vi "customise_left_slider.vi"(8 "error in":errorcluster, 11 "slide_left_ref":refnum<vi>) -> (0 "error out":errorcluster)   [LabVIEW 2020]
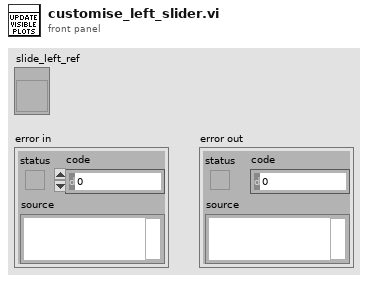
[diagram p1: front panel]
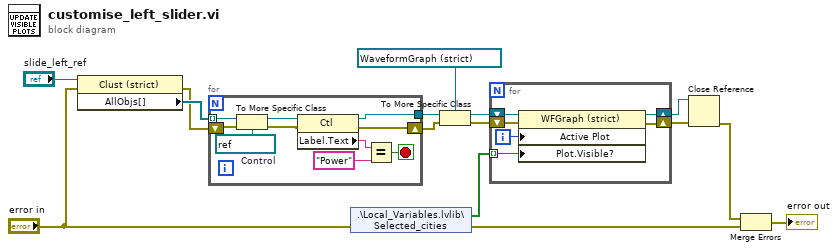
[diagram p0: block diagram]
diagram:
  n1 = property class="Clust (strict)"(reference="slide_left_ref", error in="error in") -> (error out=w2:errorcluster, "AllObjs[]"=w4:refnum<vi>[])  [unwired: 1 out]
  n2 = for {
    tunnel: w4 -> [w25] mode=indexing
    tunnel: [w19] -> w3
    shift-right: [w16] -> w1
    shift-left: w2 -> [w18]
    stop <- w20 stop-if-true
    w23 = refnum<vi> refnum  # Control
    n3 = To More Specific Class(target class=w23, reference=w25, error in=w18) -> (specific class reference=w24:refnum<vi>, error out=w17:errorcluster)
    n4 = property class="Ctl"(reference=w24, error in=w17) -> (reference out=w19:refnum<vi>, error out=w16:errorcluster, "Label.Text"=w22:string)
    n5 = Equal?(x=w22, y="Power") -> (x = y?=w20:bool)
  }
  n6 = shared-variable ".\\Local_Variables.lvlib\\Selected_cities"(error in="error in") -> (w15:bool[], error out=w5:errorcluster)
  n7 = To More Specific Class(target class=refnum<vi> refnum ("Power"), reference=w3, error in=w1) -> (specific class reference=w14:refnum<vi>, error out=w11:errorcluster)
  n8 = for {
    tunnel: w15 -> [w30] mode=indexing
    shift-right: [w27] -> w9
    shift-left: w14 -> [w31]
    shift-right: [w26] -> w10
    shift-left: w11 -> [w28]
    i -> [w29]
    n9 = property class="WFGraph (strict)"(reference=w31, error in=w28, "Active Plot"=w29, "Plot.Visible?"=w30) -> (reference out=w27:refnum<vi>, error out=w26:errorcluster)
  }
  n10 = Close Reference(reference=w9, error in (no error)=w10) -> (error out=w8:errorcluster)
  n11 = Merge Errors(w8, w5) -> (→"error out":errorcluster)
